vi "transmitOnly.vi"() -> ()   [LabVIEW 2023]
uses:
  <vilib>/DAQmx/write.llb/DAQmx Write (Analog Wfm 1Chan NSamp).vi
  <vilib>/DAQmx/create/channels.llb/DAQmx Create Channel (AO-Voltage-Basic).vi
  <vilib>/DAQmx/configure/timing.llb/DAQmx Timing (Sample Clock).vi
  <vilib>/DAQmx/miscellaneous.llb/DAQmx Fill In Error Info.vi
  <vilib>/measure/NI_MABase.lvlib
  <resource>/objmgr/daqmx.rc
panel:
  out "error out":errorcluster
  out "SampClk.Rate":dbl
  out "number of samples written per channel":u32
  out "Waveform Graph":waveform(dbl)(graph)
  in  "amplitude":dbl=1.0 format="%0.2p"
  in  "frequency":dbl=10.0 format="%0.2p"
  in  "samples per channel":i32=1000
  in  "fs":dbl=1000.0 format="%0.2f"
  in  "maximum value":dbl=10.0 format="%0.2f"
  in  "AO Channel Name":string="/ai1"
  in  "DAQmx Device Name":tag
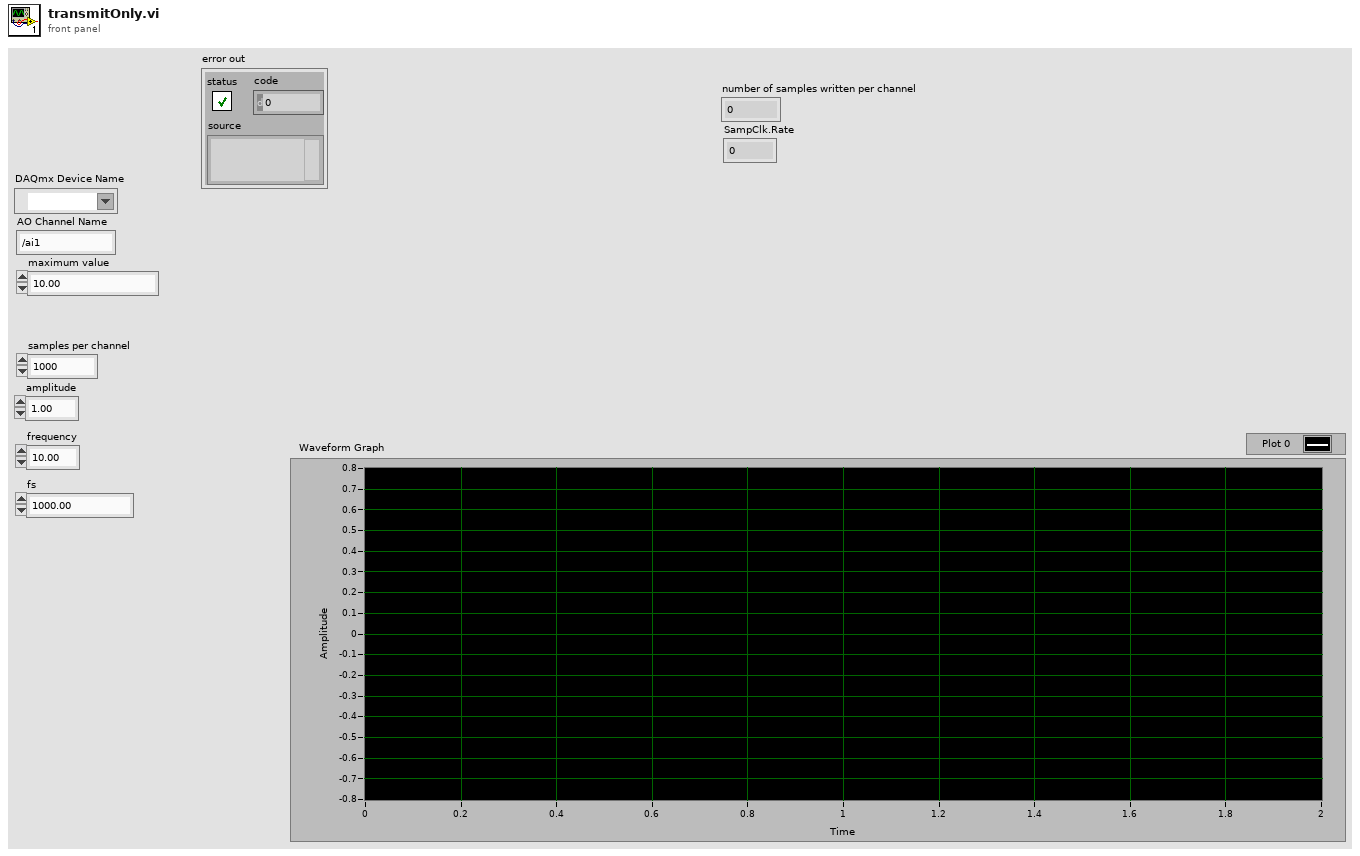
[diagram p1: front panel]
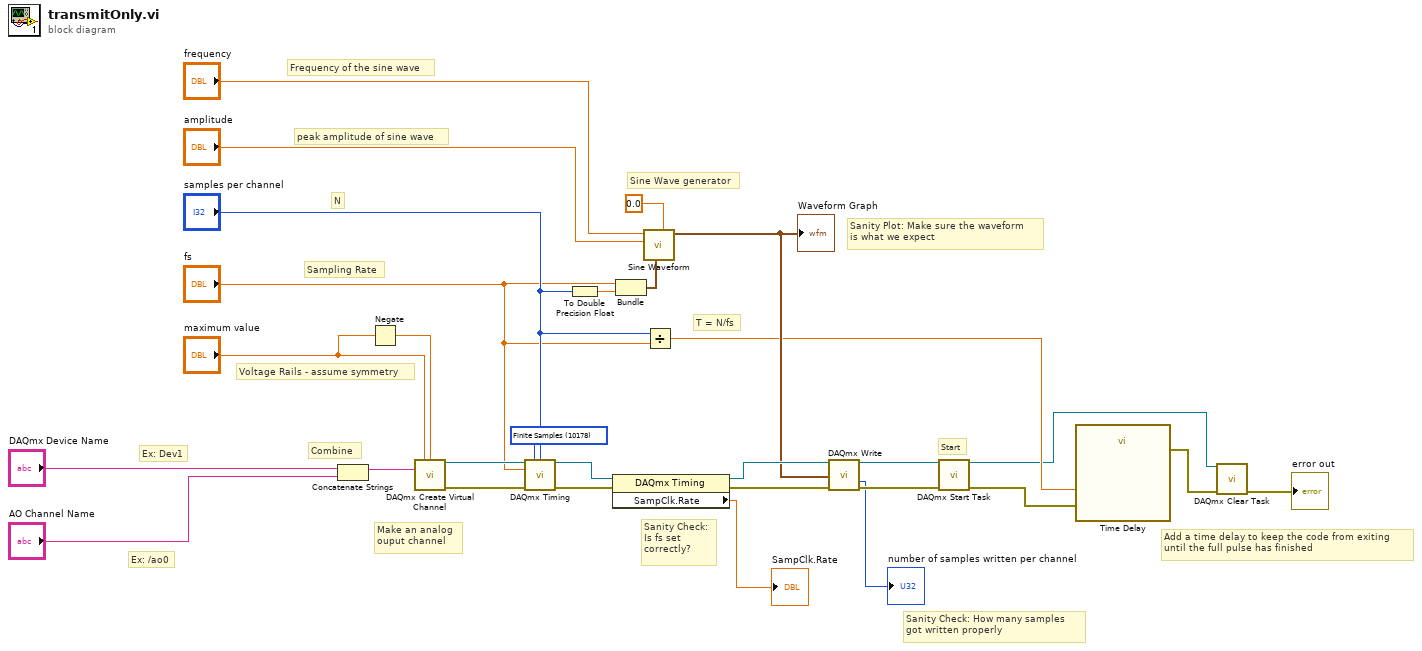
[diagram p0: block diagram]
diagram:
  w20 = 10178 items=["Finite Samples"=10178, "Continuous Samples"=10123, "Hardware Timed Single Point"=12522] ("sample mode")
  # "Add a time delay to keep the code from exiting\nuntil the full pulse has finished"
  # "Start"
  # "T = N/fs"
  # "Make an analog\nouput channel"
  # "Sanity Check: How many samples\ngot written properly"
  # "Sanity Check:\nIs fs set \ncorrectly?"
  # "Voltage Rails - assume symmetry"
  # "Sampling Rate"
  # "N"
  # "peak amplitude of sine wave"
  # "Frequency of the sine wave"
  # "Sanity Plot: Make sure the waveform\nis what we expect"
  # "Sine Wave generator"
  # "Ex: Dev1"
  # "Ex: /ao0"
  # "Combine"
  n1 = Concatenate Strings("DAQmx Device Name", "AO Channel Name") -> (w27:string)
  n2 = Negate(x="maximum value") -> (-x=w21:dbl)
  n3 = call-poly <vilib>:"DAQmx Create Virtual Channel.vi"("maximum value"="maximum value", "minimum value"=w21, "physical channels"=w27) -> ("task out"=w26:refnum<k21>, "error out"=w25:errorcluster)  [unwired: 11 in]
  n4 = call-poly <vilib>:"DAQmx Timing.vi"("task/channels in"=w26, "sample mode"=w20, "samples per channel"="samples per channel", "rate"="fs", "error in"=w25) -> ("task out"=w14:refnum<k21>, "error out"=w11:errorcluster)  [unwired: 9 in]
  n5 = To Double Precision Float(number="samples per channel") -> (double precision float=w16:dbl)
  n6 = property class="DAQmx Timing"(reference=w14, error in=w11) -> (reference out=w13:refnum<k21>, error out=w9:errorcluster, "SampClk.Rate"=→"SampClk.Rate":dbl)
  n7 = Bundle("fs"="fs", w16) -> (w10:cluster{"fs":dbl, dbl})  [unwired: 1 in]
  n8 = call <vilib>:"Sine Waveform.vi"("offset"=0.0, "sampling info"=w10, "amplitude"="amplitude", "frequency"="frequency") -> ("signal out"=w8:waveform(dbl))  [unwired: 6 in, 1 out]
  "Waveform Graph" <- w8
  n9 = Divide(x="samples per channel", y="fs") -> (x/y=w4:dbl)
  n10 = call-poly <vilib>:"DAQmx Write.vi"("task/channels in"=w13, "data"=w8, "error in"=w9) -> ("task out"=w24:refnum<k21>, "number of samples written per channel"=→"number of samples written per channel":u32, "error out"=w23:errorcluster)  [unwired: 10 in]
  n11 = call <vilib>:"DAQmx Start Task.vi"("task/channels in"=w24, "error in"=w23) -> ("task out"=w3:refnum<k21>, "error out"=w7:errorcluster)  [unwired: 12 in]
  n12 = call "Time Delay"("error in (no error)"=w7, "Delay Time (s)"=w4) -> ("error out"=w2:errorcluster)  [unwired: 9 in]
  n13 = call <vilib>:"DAQmx Clear Task.vi"("task in"=w3, "error in"=w2) -> ("error out"=→"error out":errorcluster)  [unwired: 13 in]
